vi "AssignAndCount60.vi"(6 "Last region":bool=TRUE, 7 "Photon counter area 1 in":u16, 8 "Last laser bit in":bool, 9 "PMT bits in":bool[](array[boolean])=[FALSE, FALSE, FALSE, FALSE, FALSE, FALSE, FALSE, FALSE, FALSE, FALSE, FALSE, FALSE, FALSE, FALSE, FALSE, FALSE, FALSE, FALSE, FALSE, FALSE, FALSE, FALSE, FALSE, FALSE, FALSE, FALSE, FALSE, FALSE, FALSE, FALSE, FALSE, FALSE, FALSE, FALSE, FALSE, FALSE, FALSE, FALSE, FALSE, FALSE, FALSE, FALSE, FALSE, FALSE, FALSE, FALSE, FALSE, FALSE, FALSE, FALSE, FALSE, FALSE, FALSE, FALSE, FALSE, FALSE, FALSE, FALSE, FALSE, FALSE], 10 "Laser bits in":bool[](array[boolean])=[FALSE, FALSE, FALSE, FALSE, FALSE, FALSE, FALSE, FALSE, FALSE, FALSE, FALSE, FALSE, FALSE, FALSE, FALSE, FALSE, FALSE, FALSE, FALSE, FALSE, FALSE, FALSE, FALSE, FALSE, FALSE, FALSE, FALSE, FALSE, FALSE, FALSE, FALSE, FALSE, FALSE, FALSE, FALSE, FALSE, FALSE, FALSE, FALSE, FALSE, FALSE, FALSE, FALSE, FALSE, FALSE, FALSE, FALSE, FALSE, FALSE, FALSE, FALSE, FALSE, FALSE, FALSE, FALSE, FALSE, FALSE, FALSE, FALSE, FALSE], 11 "Photon counter area 2 in":u16) -> (0 "New last laser bit out":bool, 3 "Photon counter area 2 out":u16, 4 "New last region out":bool, 5 "Photon counter area 1 out":u16)   [LabVIEW 2012]
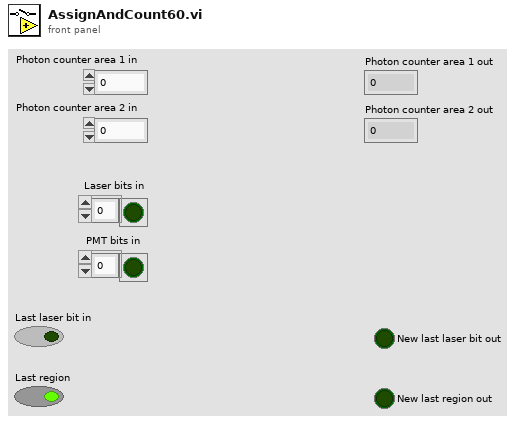
[diagram p1: front panel]
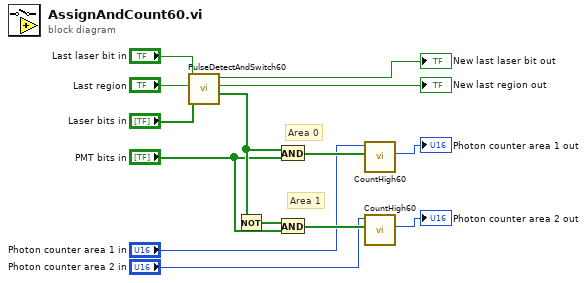
[diagram p0: block diagram]
diagram:
  # "Area 1"
  # "Area 0"
  n1 = call "PulseDetectAndSwitch60.vi"("Laser bits in"="Laser bits in", "Last region"="Last region", "Last laser bit in"="Last laser bit in") -> ("Region array out"=w11:bool[], "New last region out"=→"New last region out":bool, "New last laser bit out"=→"New last laser bit out":bool)  [unwired: 6 in]
  n2 = Not(x=w11) -> (.not. x?=w10:bool[])
  n3 = And(x=w11, y="PMT bits in") -> (x .and. y?=w8:bool[])
  n4 = And(x=w10, y="PMT bits in") -> (x .and. y?=w7:bool[])
  n5 = call "CountHigh60.vi"("60bit input"=w8, "Previous high count"="Photon counter area 1 in") -> ("New high count"=→"Photon counter area 1 out":u16)  [unwired: 9 in]
  n6 = call "CountHigh60.vi"("60bit input"=w7, "Previous high count"="Photon counter area 2 in") -> ("New high count"=→"Photon counter area 2 out":u16)  [unwired: 9 in]
